vi "Get DDG Optical Width Enabled.vi"(11 "puiEnabled":u32) -> (2 "function return":u32, 3 "puiEnabled out":u32)   [LabVIEW 2018, in "AndorSDK.lvlib"]
doc: "EXPNETTYPE unsigned int WINAPI GetDDGOpticalWidthEnabled(at_u32 * puiEnabled);"
uses:
  AndorSDK.lvlib
  ATMCD32D.dll
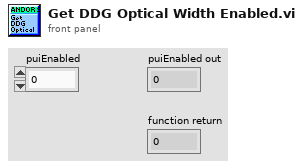
[diagram p1: front panel]
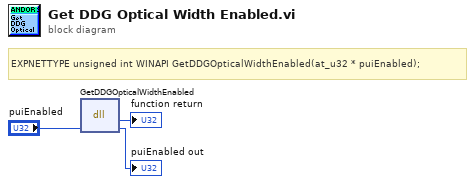
[diagram p0: block diagram]
diagram:
  # "EXPNETTYPE unsigned int WINAPI GetDDGOpticalWidthEnabled(at_u32 * puiEnabled);"
  n1 = dll-call lib="PTH2babs E\nPersönliches02 - Arbeit03-HiwijobsLabviewCodelibANDOR\tAndor SDK\nATMCD32D.*" fn="GetDDGOpticalWidthEnabled"("puiEnabled"="puiEnabled") -> (→"function return":u32, "puiEnabled"=→"puiEnabled out":u32)  [unwired: 3 in, 2 out]
